vi "set_absolute_class_path.vi"(4 "error in (no error)":errorcluster, 5 "Value":path, 6 "Container State":T2, 7 "Display State In":T1={"configuration visible?"=TRUE, "label visible?"=TRUE, "settings visible?"=TRUE, "start path"=path ""}) -> (0 "error out":errorcluster, 3 "Display State Out":T1={"configuration visible?"=TRUE, "label visible?"=TRUE, "settings visible?"=TRUE, "start path"=path ""})   [LabVIEW 2010, in "XComponentSpecification.xctl"]
uses:
  XComponentSpecification.xctl
  <vilib>/_xctls/Container State.ctl
  state.ctl
  data.ctl
  <vilib>/_xctls/XControlSupport.lvlib
panel:
  # "Replace the Value Control below with a Control of desired type.\nDo not remove this Control or the others from the connector pane.\nDo not change the connector pane pattern.\nThe Value control should always be the third terminal from top on the input side in the connector pane."
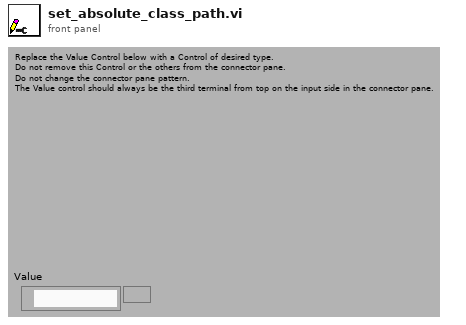
[diagram p1: front panel]
types:
  T1 = typedef "XComponentSpecification.xctl/state.ctl" = cluster{"configuration visible?":bool, "label visible?":bool, "settings visible?":bool, "start path":path}
  T2 = typedef "XControlSupport.lvlib/Container State.ctl" = cluster{"Indicator?":bool, "Run Mode?":bool, " Refnum":refnum<vi>}
  T3 = typedef "XComponentSpecification.xctl/data.ctl" = cluster{"class path":string, "configuration":string, "label":string, "settings name":string}
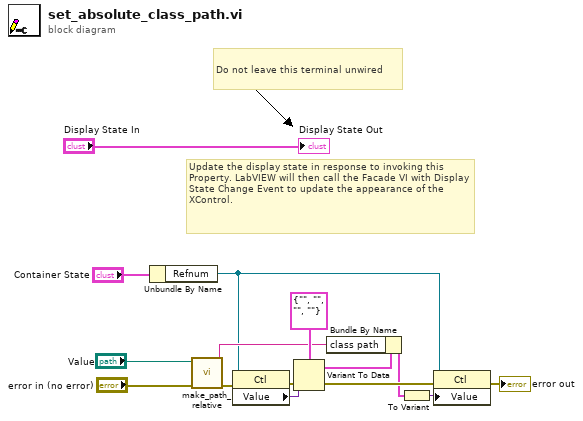
[diagram p0: block diagram]
diagram:
  # "Do not leave this terminal unwired"
  # "Update the display state in response to invoking this Property. LabVIEW will then call the Facade VI with Display State Change Event to update the appearance of the XControl."
  n1 = Unbundle By Name("Container State") -> ("Refnum"=w7:refnum<vi>)
  n2 = call "make_path_relative.vi"("error in (no error)"="error in (no error)", "absolute path"="Value") -> ("error out"=w11:errorcluster, "relative path"=w8:string)  [unwired: 8 in]
  n3 = property class="Ctl"(reference=w7, error in=w11) -> (error out=w12:errorcluster, "Value"=w13:variant)  [unwired: 1 out]
  n4 = Variant To Data(error in=w12, Variant=w13, type=T3 {"class path"="", "configuration"="", "label"="", "settings name"=""} ("component specification")) -> (error out=w6:errorcluster, data=w9:T3)
  n5 = Bundle By Name(cluster=w9, "class path"=w8) -> (w5:T3)
  n6 = To Variant(anything=w5) -> (Variant=w4:variant)
  n7 = property class="Ctl"(reference=w7, error in=w6, "Value"=w4) -> (error out=→"error out":errorcluster)  [unwired: 1 out]
  "Display State Out" <- "Display State In"
